vi "Parameter.vi"(9 "In":string, 10 "VIId":string, 11 "VariablesRef":T1) -> ()   [LabVIEW 2018, in "Dialog.lvlib"]
uses:
  Dialog.lvlib
  <userlib>/_OpenG.lib/dictionary/dictionary.llb/Dictionary Object RefNum__ogtk.ctl
  <userlib>/_OpenG.lib/dictionary/dictionary.llb/Dictionary Object RefNum - Enum__ogtk.ctl
  <vilib>/addons/_JKI.lib/Serialization/JSON/JKI JSON Serialization.lvlib
panel:
  in  "Tab Control":enum32{"Config", "控件"}(tab)
  in  "ArrayType":enum32{"AlertDialog", "ConfirmDialog"}(tab)
  in  "对话框文本_AlertDialog":string caption="对话框文本"
  in  "图片名称_AlertDialog":string(combo) caption="图片名称(Config\\Pictures)"
  in  "对话框文本_ConfirmDialog":string caption="对话框文本"
  in  "图片名称_ConfirmDialog":string(combo) caption="图片名称(Config\\Pictures)"
  in  "方法(Method)":enum16{"AlertDialog", "ConfirmDialog"}(ring)
  # "注：图片名称为空，则不显示图片"
  # "注：图片名称为空，则不显示图片"
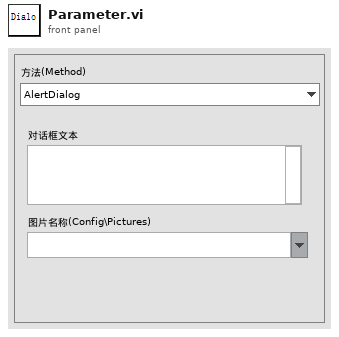
[diagram p1: front panel]
types:
  T1 = typedef "Dictionary Object RefNum__ogtk.ctl" = refnum<k1>
  T2 = cluster{"AlertDialog":cluster{"json":cluster{"Method":string, "Message":string, "PicName":string}}, "ConfirmDialog":cluster{"json":cluster{"Method":string, "Message":string, "PicName":string}}}
  T3 = enum32{"Invalid", "Standard", "Closed", "Hidden", "Minimized", "Maximized"}
  T4 = enum32{"invalid app kind", "Development System", "Run Time System", "Student Edition", "Embedded LabVIEW", "Evaluation", "Custom"}
  T5 = cluster{"Core":cluster{"Current VI Reference":refnum<vi>, "Close Panel on Exit?":bool}, "Parameter":cluster{"VariableRef":T1}, "Synchronize":cluster{"EnqueueData":cluster{"Action":enum16{"Create", "Query", "Revert", "UpdateVariable", "Close"}, "Data":variant}, "Echo":cluster{"VIRef":refnum<vi>, "JsonOut":string, "Status":string}, "Communicate":cluster{"ID":string, "JsonIn":string, "VarRef":T1}, "Queue":refnum<queue>}, "DialogClusters":cluster{"AlertDialog":cluster{"json":cluster{"Method":string, "Message":string, "PicName":string}}, "ConfirmDialog":cluster{"json":cluster{"Method":string, "Message":string, "PicName":string}}}}
  T6 = cluster{"EnqueueData":cluster{"Action":enum16{"Create", "Query", "Revert", "UpdateVariable", "Close"}, "Data":variant}, "Echo":cluster{"VIRef":refnum<vi>, "JsonOut":string, "Status":string}, "Communicate":cluster{"ID":string, "JsonIn":string, "VarRef":T1}, "Queue":refnum<queue>}
  T7 = cluster{"Current VI Reference":refnum<vi>, "Close Panel on Exit?":bool}
  T8 = cluster{"json":cluster{"Method":string, "Message":string, "PicName":string}}
  T9 = cluster{"Action":enum16{"Create", "Query", "Revert", "UpdateVariable", "Close"}, "Data":variant}
  T10 = cluster{"ID":string, "JsonIn":string, "VarRef":T1}
  T11 = enum16{"Create", "Query", "Revert", "UpdateVariable", "Close"}
  T12 = cluster{"VIRef":refnum<vi>, "JsonOut":string, "Status":string}
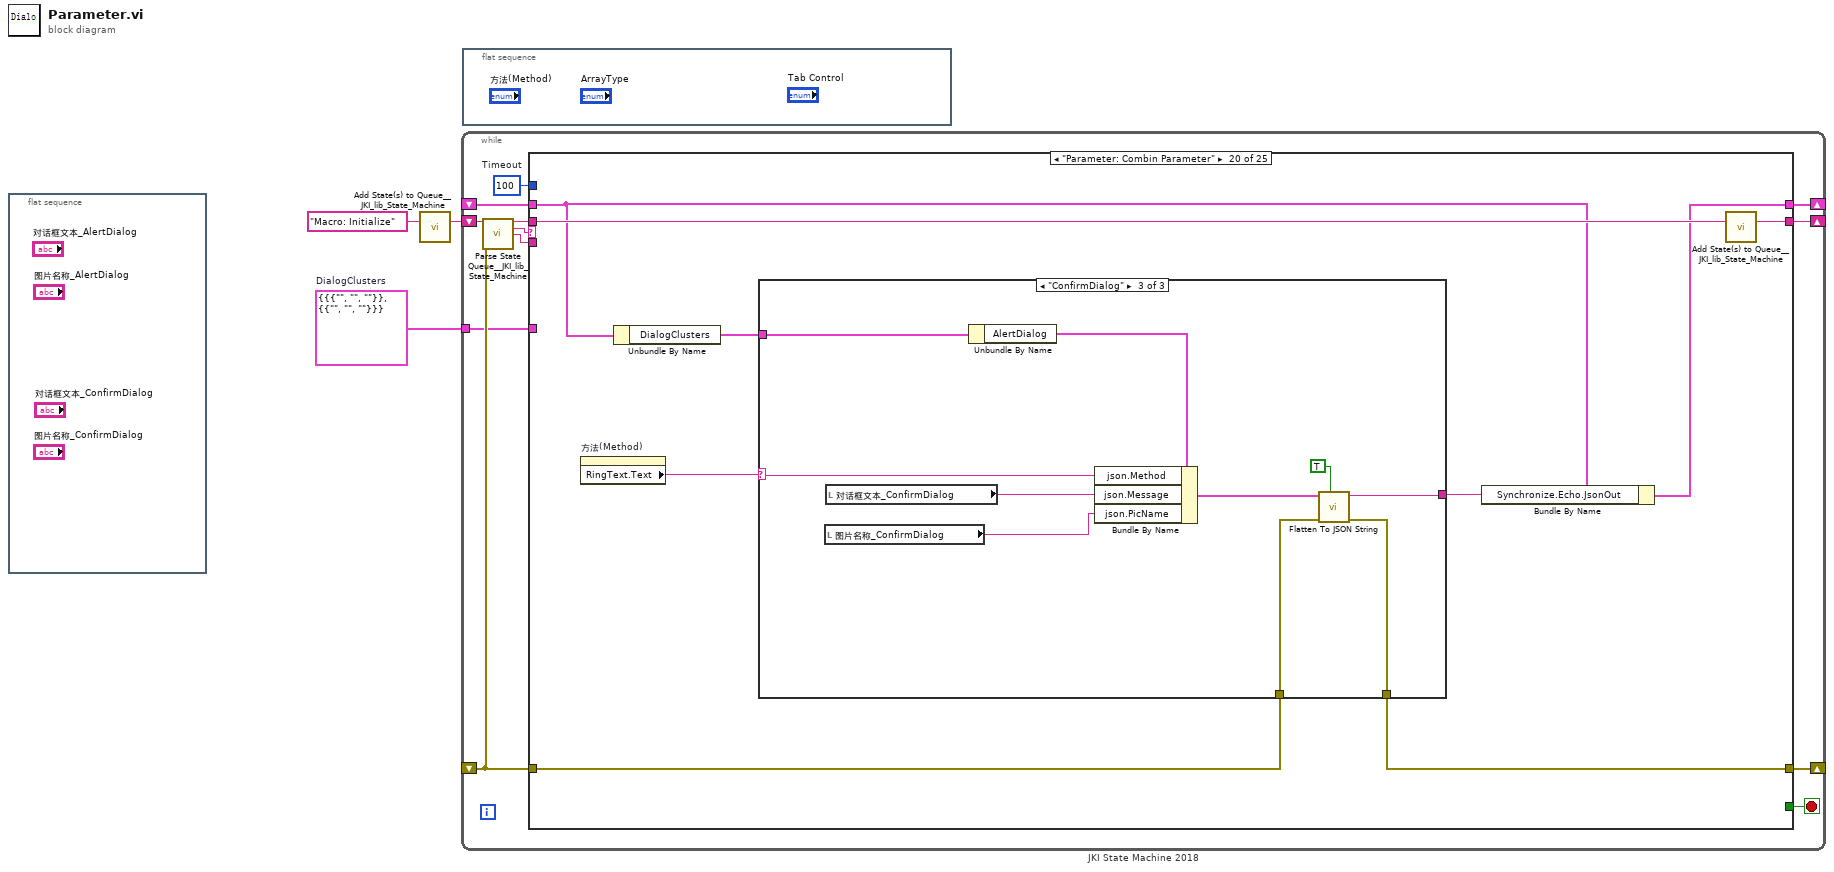
[diagram p0: block diagram]
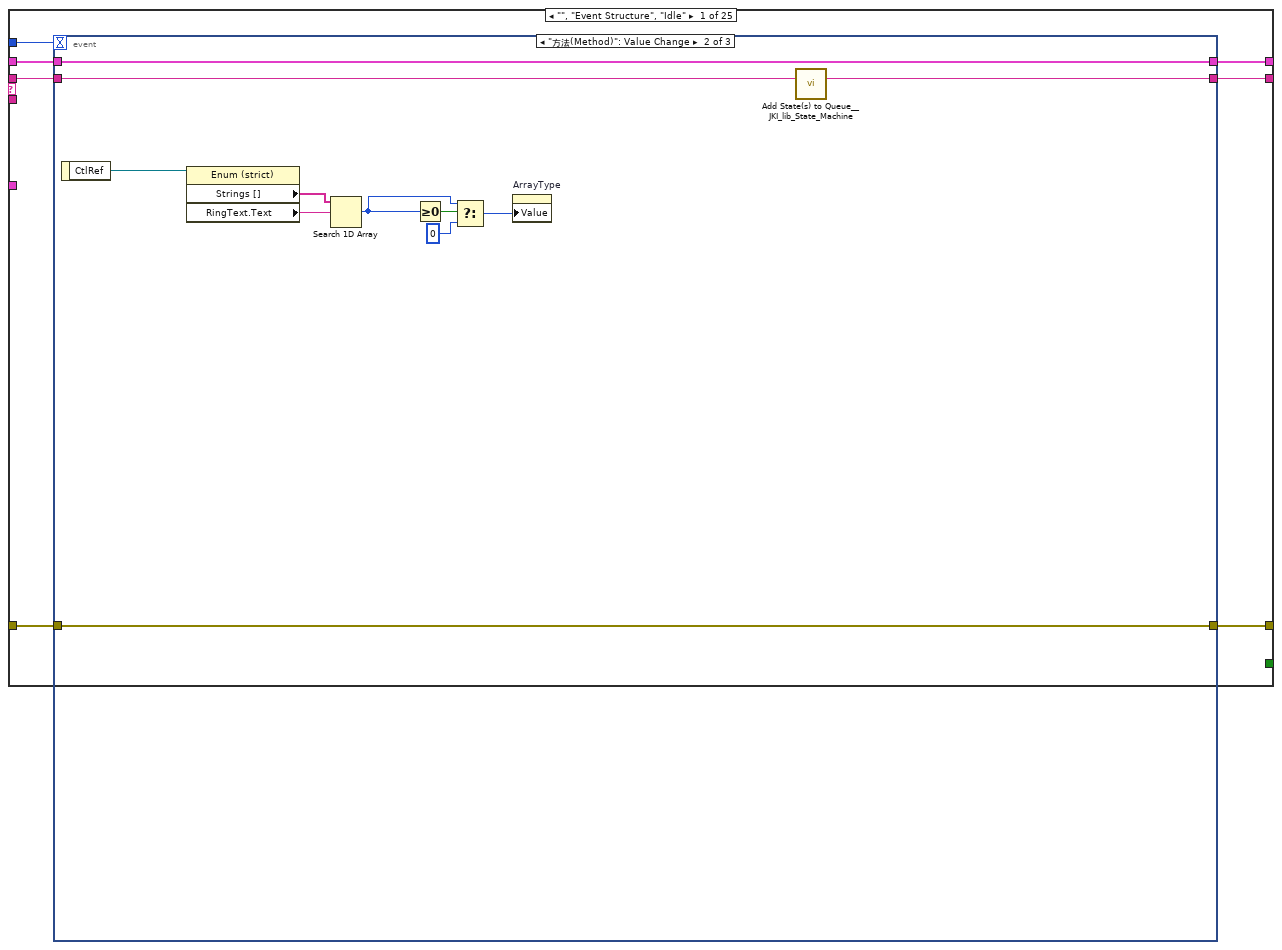
[diagram p2: hidden frame]
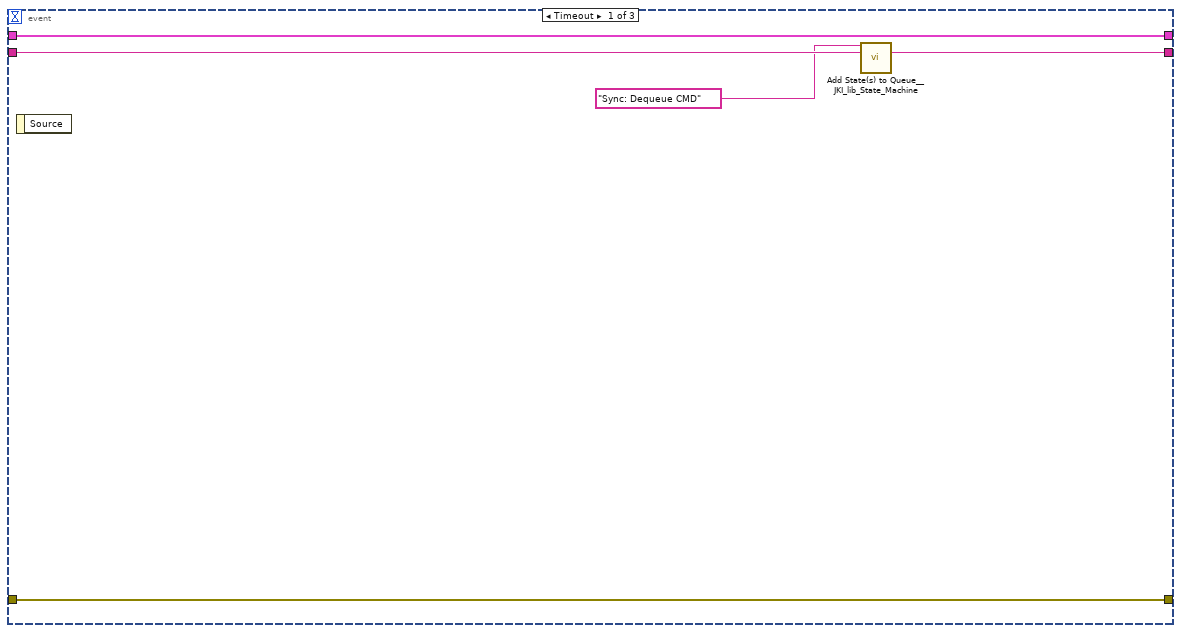
[diagram p3: hidden frame]
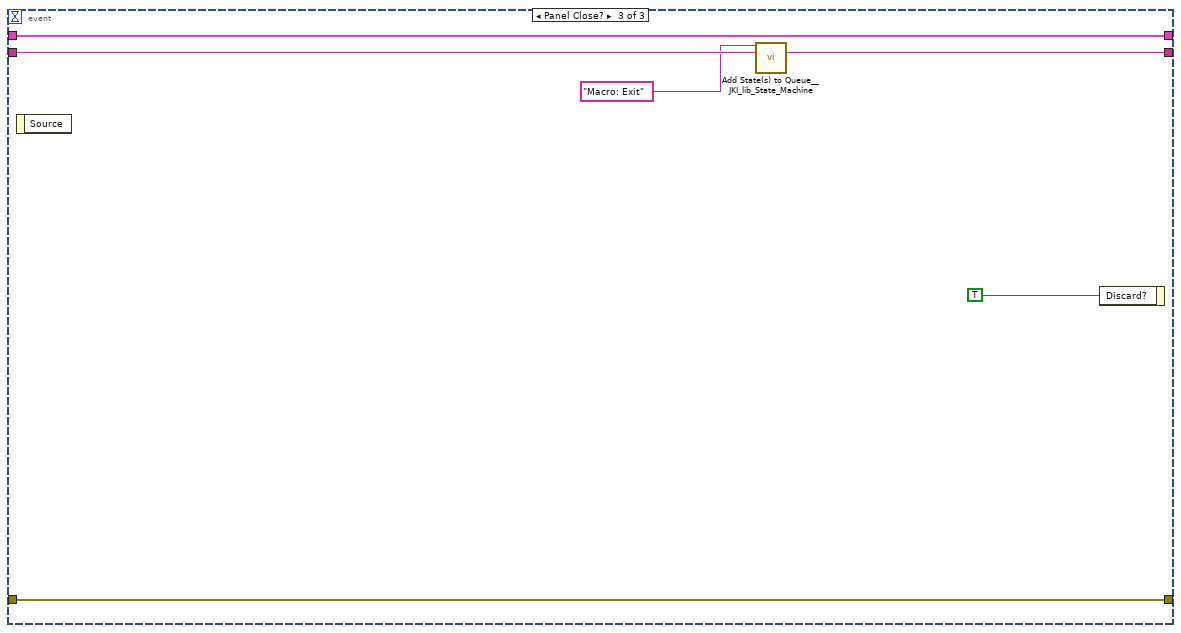
[diagram p4: hidden frame]
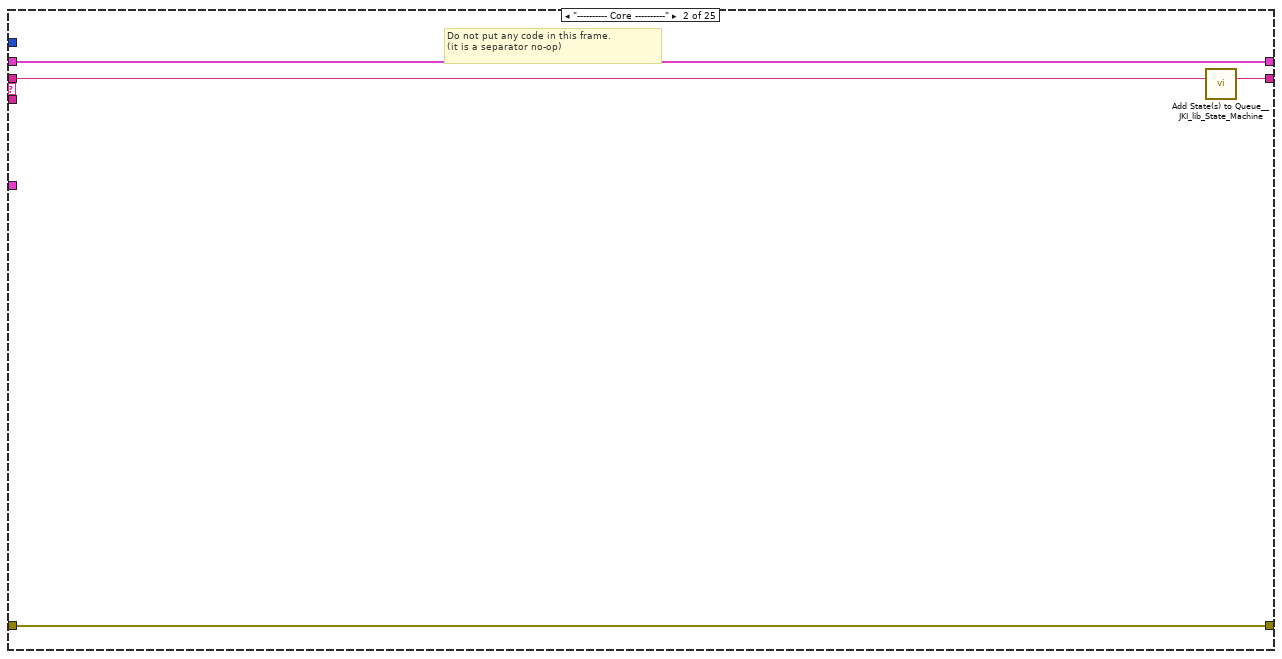
[diagram p5: hidden frame]
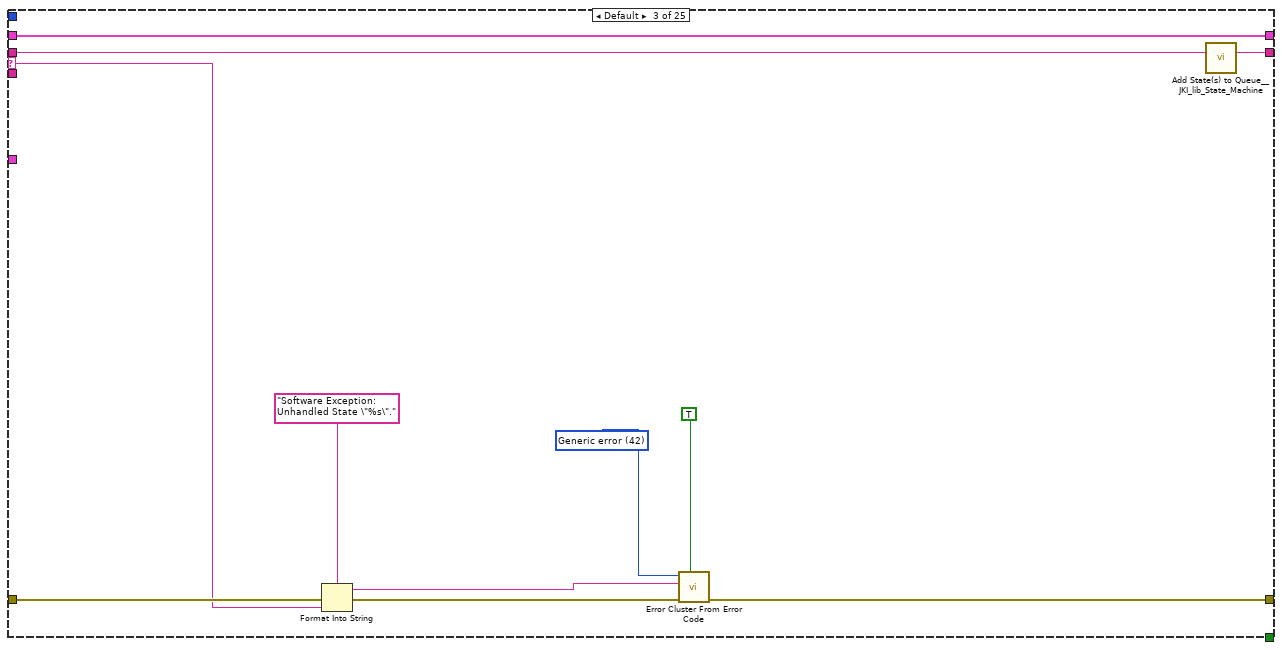
[diagram p6: hidden frame]
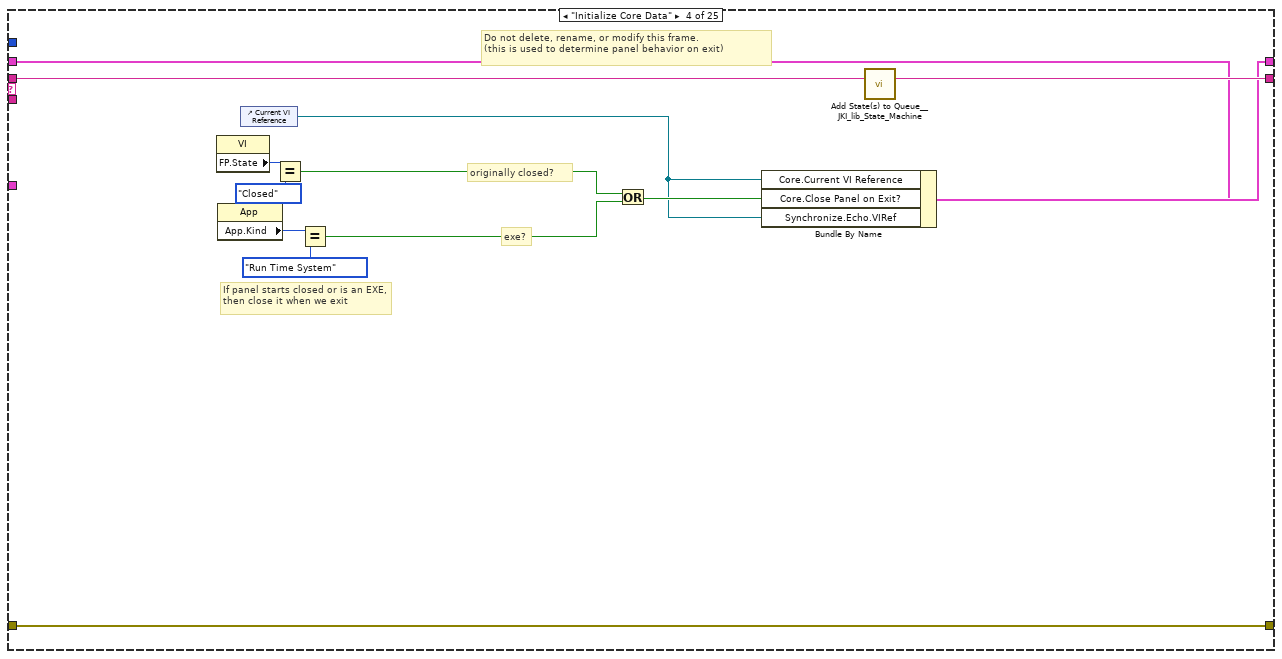
[diagram p7: hidden frame]
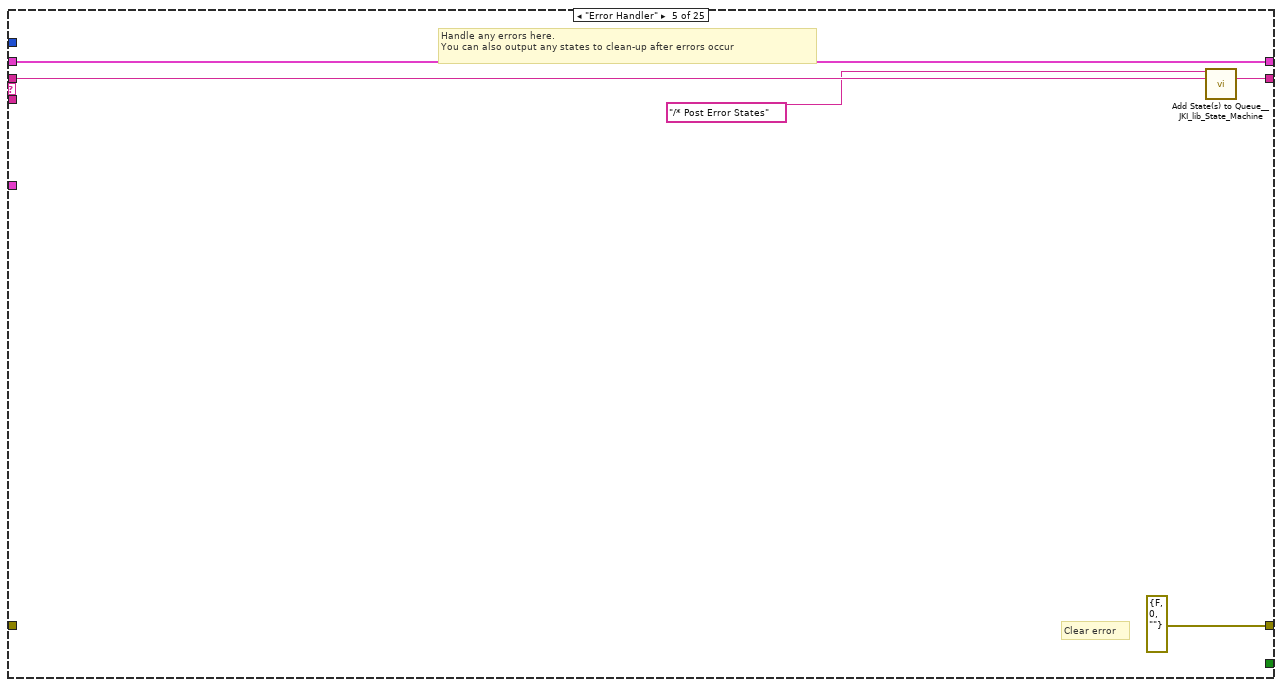
[diagram p8: hidden frame]
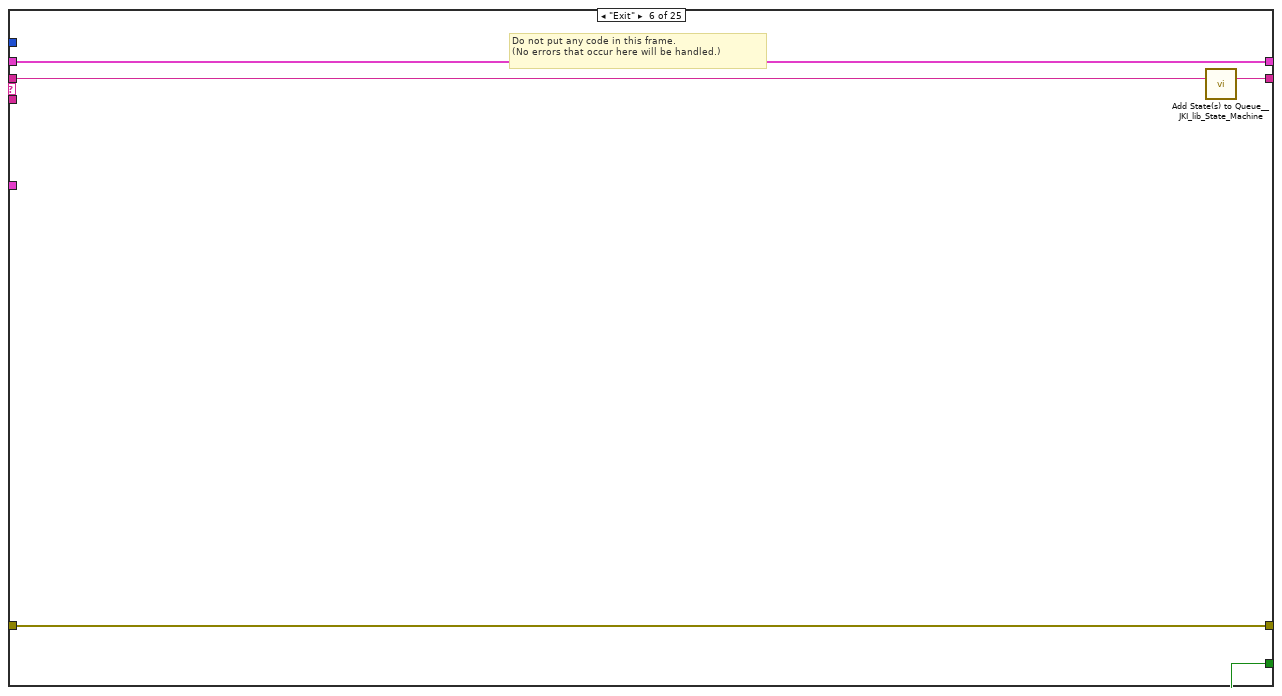
[diagram p9: hidden frame]
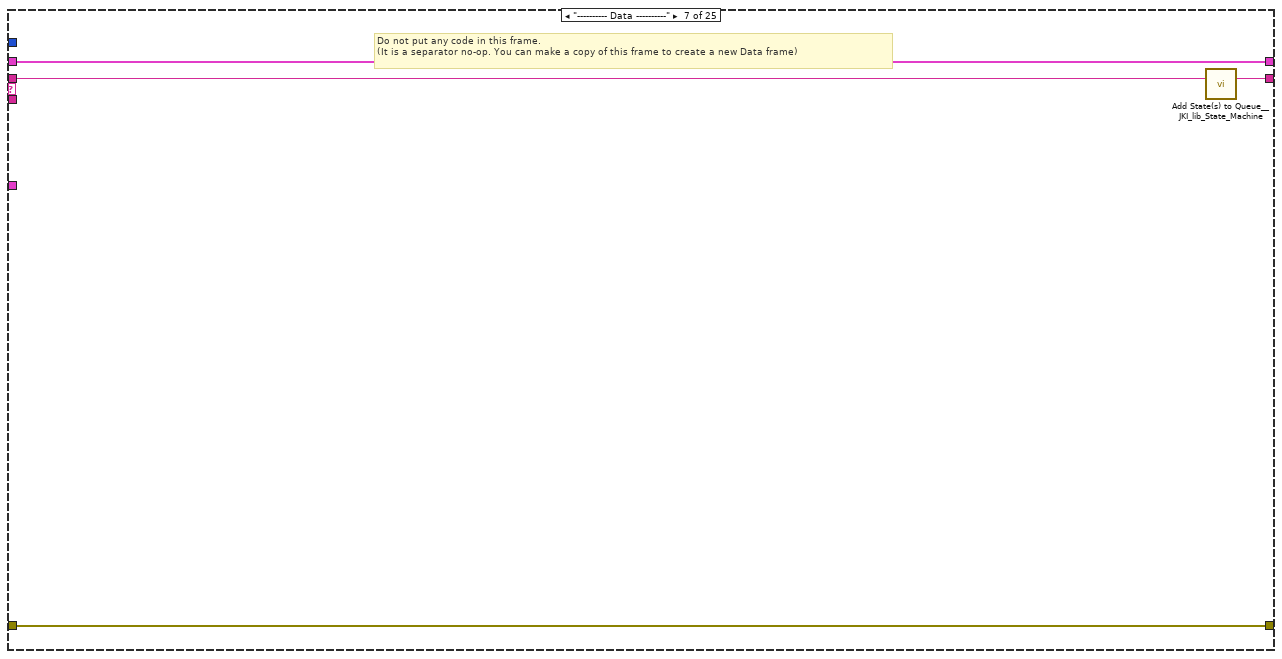
[diagram p10: hidden frame]
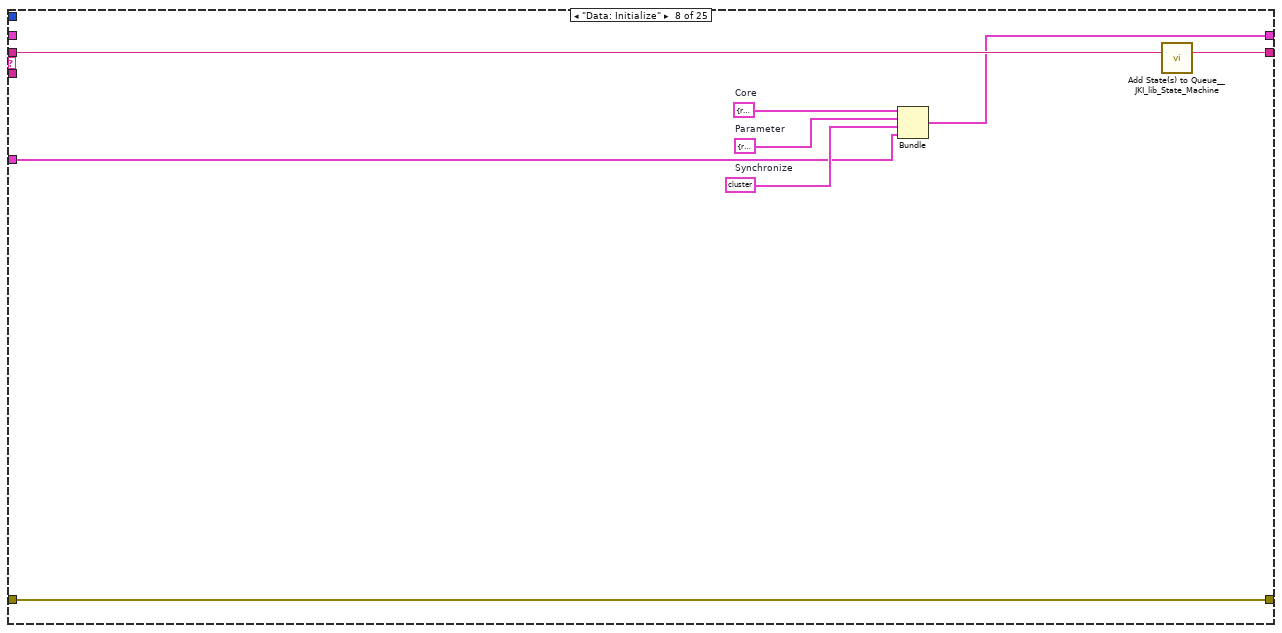
[diagram p11: hidden frame]
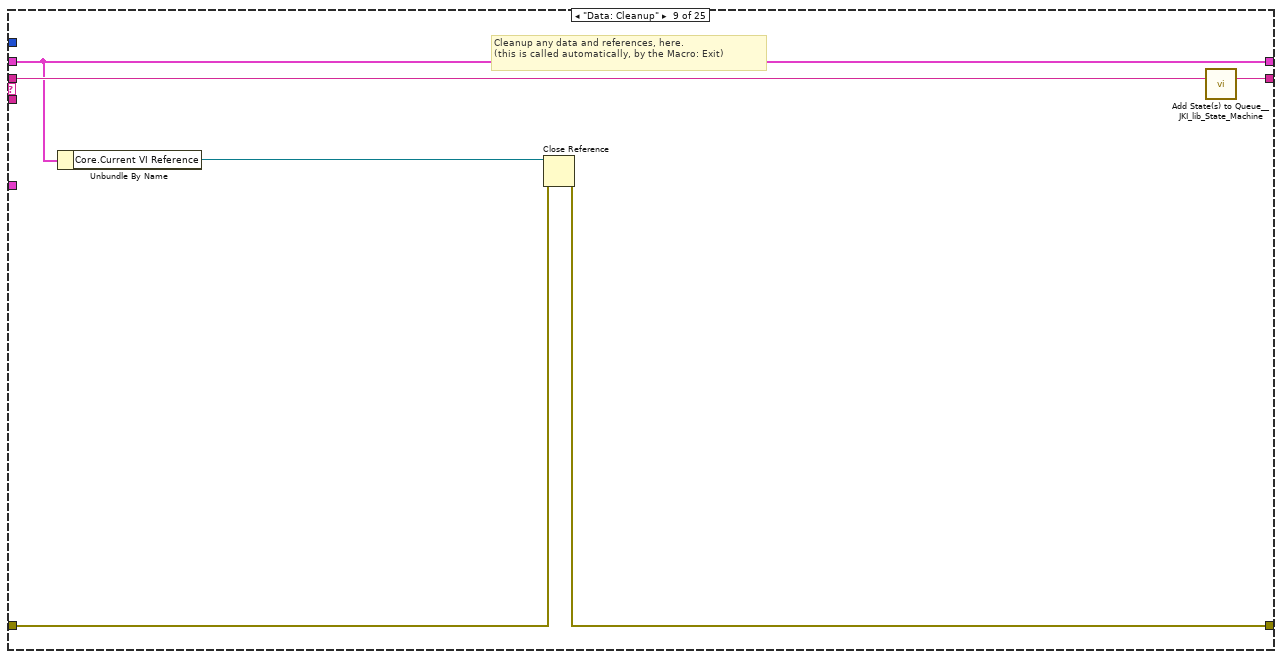
[diagram p12: hidden frame]
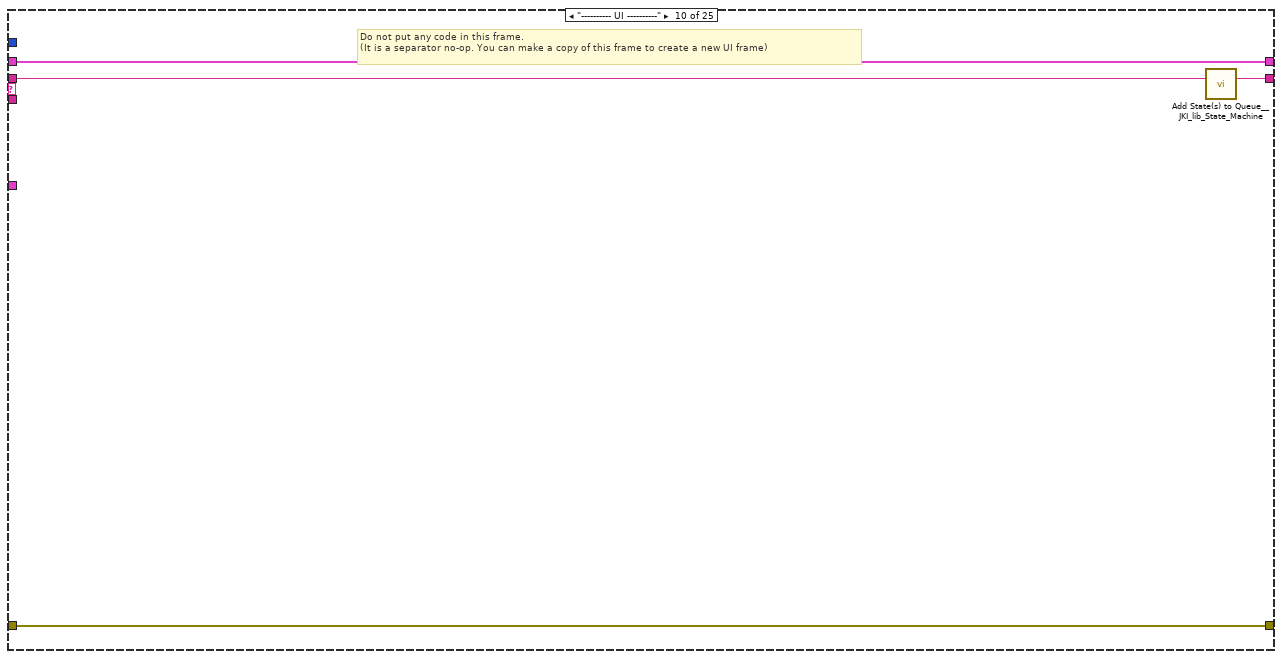
[diagram p13: hidden frame]
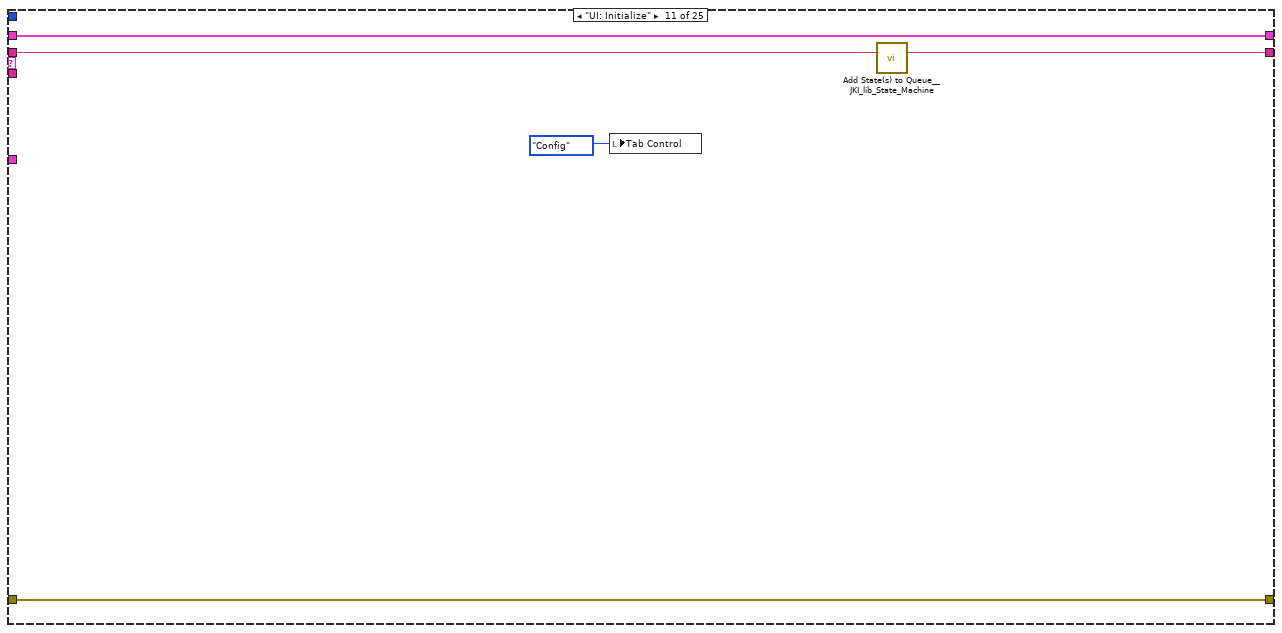
[diagram p14: hidden frame]
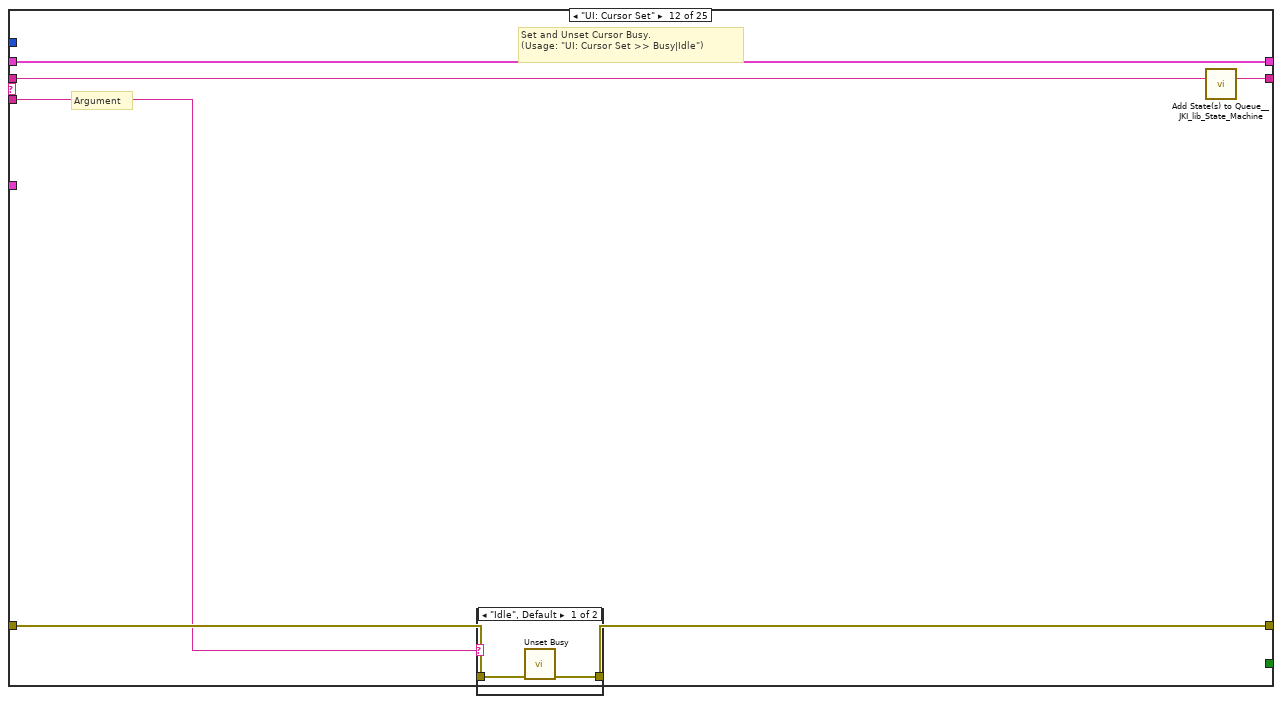
[diagram p15: hidden frame]
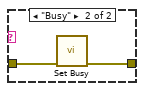
[diagram p16: hidden frame]
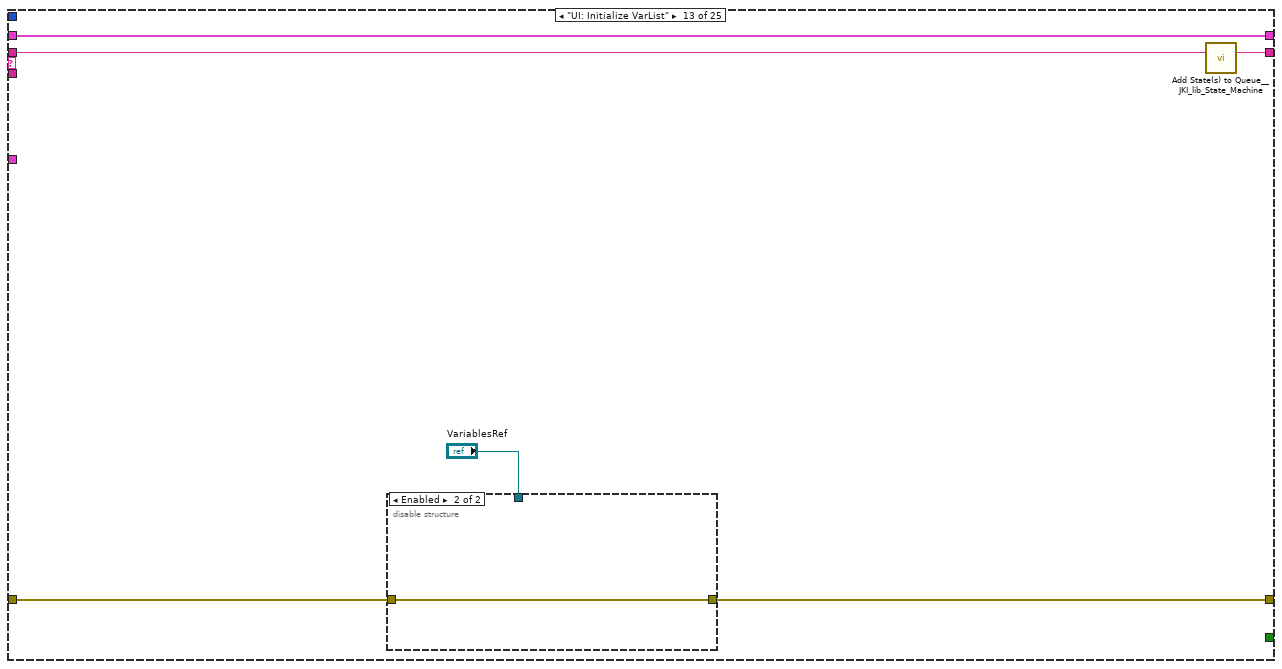
[diagram p17: hidden frame]
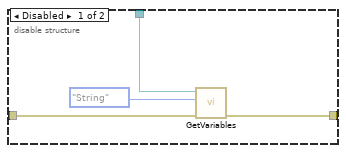
[diagram p18: hidden frame]
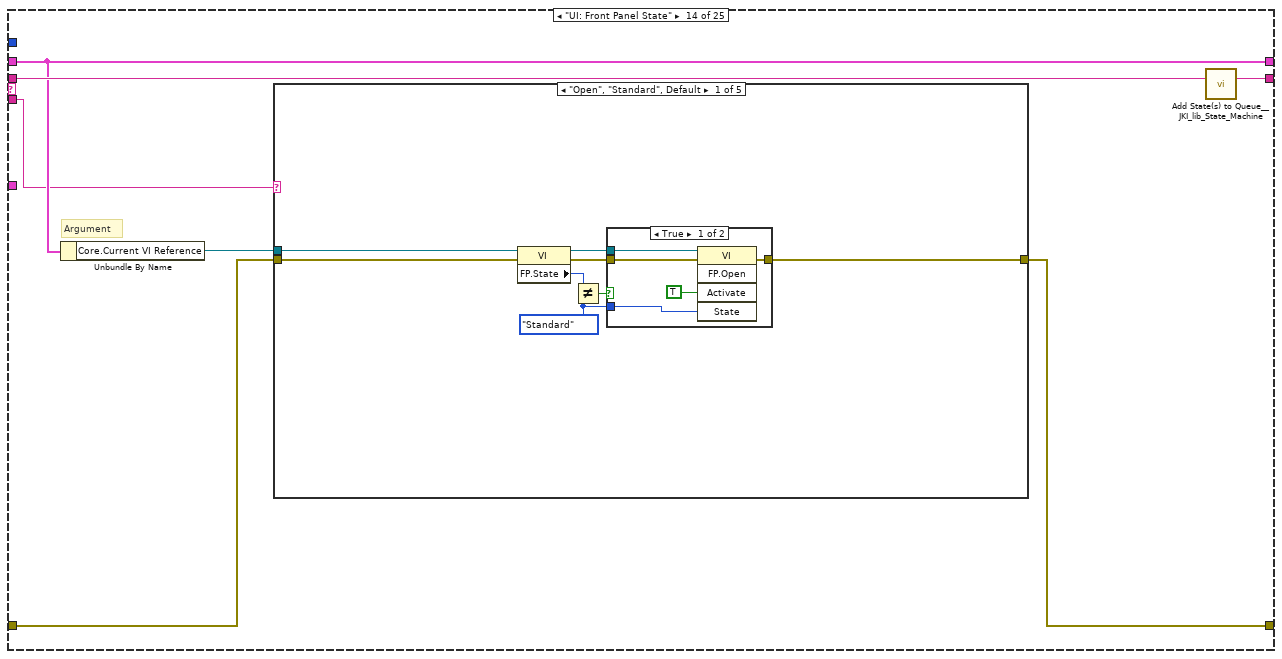
[diagram p19: hidden frame]
diagram:
  w1 = T2 {"AlertDialog"={"json"={"Method"="", "Message"="", "PicName"=""}}, "ConfirmDialog"={"json"={"Method"="", "Message"="", "PicName"=""}}}  # DialogClusters
  n1 = flat-sequence {
    frame #0 {
    }
  }
  n2 = call <vilib>:"Add State(s) to Queue__JKI_lib_State_Machine.vi"("State(s) in (\"\")"="Macro: Initialize") -> ("States Out"=w3:string)  [unwired: 14 in]
  n3 = while "JKI State Machine 2018" {
    shift-right: [w8] -> _
    shift-left: _ -> [w7]
    shift-right: [w11] -> _
    shift-left: _ -> [w5]
    shift-right: [w10] -> _
    shift-left: w3 -> [w12]
    tunnel: w1 -> [w4]
    stop <- w9 stop-if-true
    w6 = 100  # Timeout
    n4 = call <vilib>:"Parse State Queue__JKI_lib_State_Machine.vi"("State Queue"=w12, "Error In (no error)"=w5) -> ("Remaining States"=w14:string, "Current State"=w15:string, "Arguments"=w13:string)  [unwired: 11 in]
    n5 = case shown="\"Parameter: Combin Parameter\"" w15 {
      selector: w15 -> [_ _ w49 _ _ _ _ _ _ _ _ _ _ _ _ _ _ _ _ _ _ _ _ _ _]
      tunnel: w14 -> [w22 w48 w53 w72 w77 w82 w86 w94 w100 w104 w109 w115 w125 w137 w206 w211 w221 w225 w233 w280 w305 w314 w329 w373 w388]
      tunnel: w13 -> [_ _ _ _ _ _ _ _ _ _ _ w110 _ w131 _ _ _ _ _ _ _ _ _ _ _]
      tunnel: w7 -> [w20 w45 w51 w65 w74 w80 w83 _ w95 w101 w106 w113 w123 w133 w203 w208 w218 w222 w228 w273 w302 w307 w327 w370 w377]
      tunnel: [w19 w46 w55 w69 errorcluster {"status"=FALSE, "code"=0, "source"=""} ("error out") w79 w84 w92 w96 w102 w105 w111 w120 w134 w204 w209 w219 w223 w229 w277 w303 w311 w316 w368 w375] -> w11
      tunnel: w5 -> [w18 w46 w54 w69 _ w79 w84 w92 w97 w102 w105 w112 w121 w135 w204 w209 w219 w223 w230 w276 w303 w312 w325 w369 w376]
      tunnel: [w21 w47 w52 w71 w76 w81 w85 w93 w99 w103 w108 w114 w124 w136 w205 w210 w220 w224 w232 w279 w304 w313 w328 w372 w387] -> w10
      tunnel: [_ _ _ _ _ TRUE _ _ _ _ _ _ _ _ _ _ _ _ _ _ _ _ _ _ _] -> w9
      tunnel: [w17 w45 w51 w70 w74 w80 w83 w89 w95 w101 w106 w113 w123 w133 w203 w208 w218 w222 w228 w278 w302 w309 w318 w370 w377] -> w8
      tunnel: w6 -> [w16 _ _ _ _ _ _ _ _ _ _ _ _ _ _ _ _ _ _ _ _ _ _ _ _]
      tunnel: w4 -> [_ _ _ _ _ _ _ w87 _ _ _ _ _ _ _ _ _ _ _ _ _ _ _ _ _]
      frame "", "Event Structure", "Idle" {
        n6 = event shown="[1] \"方法(Method)\": Value Change" {
          selector: _ -> [_ _ _]
          dyn-events: _ -> [_ _ _]
          timeout: w16 -> [_ _ _]
          tunnel: w22 -> [w27 w38 w44]
          tunnel: [w26 w37 w43] -> w21
          tunnel: w20 -> [w24 w35 w41]
          tunnel: [w25 w36 w42] -> w19
          tunnel: w18 -> [w25 w36 w42]
          tunnel: [w24 w35 w41] -> w17
          event Timeout {
            n7 = event-data() -> ()  [unwired: 1 in, 1 out]
            n8 = call <vilib>:"Add State(s) to Queue__JKI_lib_State_Machine.vi"("State(s) in Front (\"\")"="Sync: Dequeue CMD" ("State(s) in Front (\"\")"), "State(s) in (\"\")"=w27) -> ("States Out"=w26:string)  [unwired: 13 in]
          }
          event "方法(Method)": Value Change {
            n9 = event-data() -> ("CtlRef"=w31:refnum<vi>)  [unwired: 1 in]
            n10 = property class="Enum (strict)"(reference=w31) -> ("Strings []"=w30:string[], "RingText.Text"=w29:string)  [unwired: 1 in, 2 out]
            n11 = Search 1D Array(1D array=w30, element=w29) -> (index of element=w33:i32)  [unwired: 1 in]
            n12 = Greater Or Equal To 0?(x=w33) -> (x >= 0?=w34:bool)
            n13 = Select(t=w33, s=w34, f=0) -> (s? t:f=w28:i32)
            n14 = property on="ArrayType" class="TabCtl (strict)"("Value"=w28) -> ()  [unwired: 2 in, 2 out]
            n15 = call <vilib>:"Add State(s) to Queue__JKI_lib_State_Machine.vi"("State(s) in (\"\")"=w38) -> ("States Out"=w37:string)  [unwired: 14 in]
          }
          event Panel Close? {
            n16 = event-data() -> ()  [unwired: 1 in, 1 out]
            n17 = call <vilib>:"Add State(s) to Queue__JKI_lib_State_Machine.vi"("State(s) in Front (\"\")"="Macro: Exit", "State(s) in (\"\")"=w44) -> ("States Out"=w43:string)  [unwired: 13 in]
            n18 = event-data("Discard?"=TRUE) -> ()  [unwired: 1 in, 1 out]
          }
        }
      }
      frame "---------- Core ----------" {
        # "Do not put any code in this frame.\n(it is a separator no-op)"
        n19 = call <vilib>:"Add State(s) to Queue__JKI_lib_State_Machine.vi"("State(s) in (\"\")"=w48) -> ("States Out"=w47:string)  [unwired: 14 in]
      }
      frame Default {
        w58 = 42 items=["No error", "Argument error", "Memory is full", "Out of zone", "End of file", "File already open", "Generic file I/O error", "File not found", "File permission error", "Disk is full", "Duplicate path", "Too many files open", "System feature not enabled", "Resource file not found", "Cannot add resource", "Resource not found", "Image not found", "Image memory error", "Pen does not exist", "Config type invalid", "Config token not found", "Config parse error", "Config memory error", "Bad external code format", "Bad external code offset", "External code not present", "Null window", "Destroy window error", "Null menu", "Print aborted", "Bad print record", "Print driver error", "Windows error during printing", "Memory error during printing", "Print dialog error", "Generic print error", "Invalid device refnum", "Device not found", "Device parameter error", "Device unit error", "Cannot open device", "Device call aborted", "Generic error", "Cancelled by user", "Object ID too low", "Object ID too high", "Object not in heap", "Unknown heap", "Unknown object (invalid DefProc)", "Unknown object (DefProc not in table)", "Message out of range", "Invalid (null) method", "Unknown message", "Manager call not supported", "Bad address", "Network operation in progress", "Network operation timed out", "Connection is busy", "Network attribute not supported", "Network error", "Address in use", "System out of memory", "Connection aborted", "Connection refused", "Not connected", "Already connected", "Connection closed", "Initialization error (interapplication manager)", "Bad occurrence", "Wait on unbound occurrence handler", "Occurrence queue overflow", "Datalog type conflict", "Unused", "Unrecognized type (interapplication manager)", "Memory corrupt", "Failed to make temporary DLL", "Old CIN version", "Drag socket not found", "Failed to load drop-object", "Failed to register OLE object", "Failed to release OLE object", "Format specifier type mismatch", "Unknown format specifier", "Too few format specifiers", "Too many format specifiers", "Scan failed", "Newer CIN version", "Error converting to variant", "Runtime menu error", "Password tampered", "Variant attribute not found", "Incompatible variant data type", "Event data is not available", "Event Store is not present", "Occurrence is not found", "Event Queue is not created", "Event info is not available", "Refnum passed is NULL", "Error retrieving Class GUID", "Error retrieving CoClass GUID", "Error retrieving TypeLib GUID.", "Bad built application magic bytes.", "Specific driver is different from the specific driver associated with the Logical Name.", "There is no session opened to the class driver.", "Max Error", "MAX - Error with config objects", "MAX - Error loading configuration", "MAX - Group not supported"]
        n20 = Format Into String(format string="Software Exception: Unhandled State \"%s\"." ("message"), error in=w54, w49) -> (resulting string=w57:string, error out=w56:errorcluster)  [unwired: 1 in]
        n21 = call <vilib>:"Error Cluster From Error Code.vi"("show call chain? (False)"=TRUE, "error in (no error)"=w56, "error message (\"\")"=w57, "error code (0)"=w58) -> ("error out"=w55:errorcluster)  [unwired: 5 in]
        n22 = call <vilib>:"Add State(s) to Queue__JKI_lib_State_Machine.vi"("State(s) in (\"\")"=w53) -> ("States Out"=w52:string)  [unwired: 14 in]
      }
      frame "Initialize Core Data" {
        # "Do not delete, rename, or modify this frame.\n(this is used to determine panel behavior on exit)"
        # "originally closed?"
        # "exe?"
        # "If panel starts closed or is an EXE, then close it when we exit"
        n23 = property class="VI"() -> ("FP.State"=w63:T3)  [unwired: 2 in, 2 out]
        n24 = property class="App"() -> ("App.Kind"=w68:T4)  [unwired: 2 in, 2 out]
        n25 = control-ref of="Current VI Reference"() -> (w60:refnum<vi>)
        n26 = Equal?(x=w63, y=T3."Closed" ("Front Panel Window:State")) -> (x = y?=w61:bool)
        n27 = Equal?(x=w68, y=T4."Run Time System" ("Application:Kind")) -> (x = y?=w66:bool)
        n28 = Or(x=w61, y=w66) -> (x .or. y?=w64:bool)
        n29 = Bundle By Name(cluster=w65, "Core.Current VI Reference"=w60, "Core.Close Panel on Exit?"=w64, "Synchronize.Echo.VIRef"=w60) -> (w70:T5)
        n30 = call <vilib>:"Add State(s) to Queue__JKI_lib_State_Machine.vi"("State(s) in (\"\")"=w72) -> ("States Out"=w71:string)  [unwired: 14 in]
      }
      frame "Error Handler" {
        # "Handle any errors here.\nYou can also output any states to clean-up after errors occur"
        # "Clear error"
        n31 = call <vilib>:"Add State(s) to Queue__JKI_lib_State_Machine.vi"("State(s) in Front (\"\")"="/* Post Error States", "State(s) in (\"\")"=w77) -> ("States Out"=w76:string)  [unwired: 13 in]
      }
      frame "Exit" {
        # "Do not put any code in this frame.\n(No errors that occur here will be handled.)"
        n32 = call <vilib>:"Add State(s) to Queue__JKI_lib_State_Machine.vi"("State(s) in (\"\")"=w82) -> ("States Out"=w81:string)  [unwired: 14 in]
      }
      frame "---------- Data ----------" {
        # "Do not put any code in this frame.\n(It is a separator no-op. You can make a copy of this frame to create a new Data frame)"
        n33 = call <vilib>:"Add State(s) to Queue__JKI_lib_State_Machine.vi"("State(s) in (\"\")"=w86) -> ("States Out"=w85:string)  [unwired: 14 in]
      }
      frame "Data: Initialize" {
        w88 = cluster{"VariableRef":T1} {"VariableRef"=refnum}  # Parameter
        w90 = T6 {"EnqueueData"={"Action"=enum."Create", "Data"=variant}, "Echo"={"VIRef"=refnum, "JsonOut"="", "Status"=""}, "Communicate"={"ID"="", "JsonIn"="", "VarRef"=refnum}, "Queue"=refnum}  # Synchronize
        w91 = T7 {"Current VI Reference"=refnum, "Close Panel on Exit?"=FALSE}  # Core
        n34 = Bundle("Core"=w91, "Parameter"=w88, "Synchronize"=w90, "DialogClusters"=w87) -> (w89:T5)  [unwired: 1 in]
        n35 = call <vilib>:"Add State(s) to Queue__JKI_lib_State_Machine.vi"("State(s) in (\"\")"=w94) -> ("States Out"=w93:string)  [unwired: 14 in]
      }
      frame "Data: Cleanup" {
        # "Cleanup any data and references, here.\n(this is called automatically, by the Macro: Exit)"
        n36 = Unbundle By Name(w95) -> ("Core.Current VI Reference"=w98:refnum<vi>)
        n37 = Close Reference(reference=w98, error in (no error)=w97) -> (error out=w96:errorcluster)
        n38 = call <vilib>:"Add State(s) to Queue__JKI_lib_State_Machine.vi"("State(s) in (\"\")"=w100) -> ("States Out"=w99:string)  [unwired: 14 in]
      }
      frame "---------- UI ----------" {
        # "Do not put any code in this frame.\n(It is a separator no-op. You can make a copy of this frame to create a new UI frame)"
        n39 = call <vilib>:"Add State(s) to Queue__JKI_lib_State_Machine.vi"("State(s) in (\"\")"=w104) -> ("States Out"=w103:string)  [unwired: 14 in]
      }
      frame "UI: Initialize" {
        n40 = local write "Tab Control"(enum32{"Config", "控件"}."Config" ("Tab Control")) -> ()
        n41 = call <vilib>:"Add State(s) to Queue__JKI_lib_State_Machine.vi"("State(s) in (\"\")"=w109) -> ("States Out"=w108:string)  [unwired: 14 in]
      }
      frame "UI: Cursor Set" {
        # "Argument"
        # "Set and Unset Cursor Busy.\n(Usage: \"UI: Cursor Set >> Busy|Idle\")"
        n42 = case shown="\"Idle\", Default" w110 {
          tunnel: w112 -> [w117 w119]
          tunnel: [w116 w118] -> w111
          frame "Idle", Default {
            n43 = call <vilib>:"Unset Busy.vi"("error in (no error)"=w117) -> ("error out"=w116:errorcluster)  [unwired: 10 in]
          }
          frame "Busy" {
            n44 = call <vilib>:"Set Busy.vi"("error in (no error)"=w119) -> ("error out"=w118:errorcluster)  [unwired: 9 in, 1 out]
          }
        }
        n45 = call <vilib>:"Add State(s) to Queue__JKI_lib_State_Machine.vi"("State(s) in (\"\")"=w115) -> ("States Out"=w114:string)  [unwired: 14 in]
      }
      frame "UI: Initialize VarList" {
        n46 = disable-structure shown="Enabled" {
          disable-tunnel: "VariablesRef" -> [w129 _]
          disable-tunnel: w121 -> [w127 w130]
          disable-tunnel: [w126 w130] -> w120
          frame Disabled {
            n47 = call "GetVariables.vi"("error in (no error)"=w127, "VariableType"=enum16{"String", "StringArray"}."String", "DicRef"=w129) -> ("error out"=w126:errorcluster)  [unwired: 7 in, 1 out]
          }
          frame Enabled {
          }
        }
        n48 = call <vilib>:"Add State(s) to Queue__JKI_lib_State_Machine.vi"("State(s) in (\"\")"=w125) -> ("States Out"=w124:string)  [unwired: 14 in]
      }
      frame "UI: Front Panel State" {
        # "Argument"
        n49 = Unbundle By Name(w133) -> ("Core.Current VI Reference"=w132:refnum<vi>)
        n50 = case shown="\"Open\", \"Standard\", Default" w131 {
          tunnel: w135 -> [w143 w158 w169 w182 w195]
          tunnel: [w145 w159 w171 w184 w197] -> w134
          tunnel: w132 -> [w144 w156 w170 w183 w196]
          frame "Open", "Standard", Default {
            w138 = T3."Standard" ("State")
            n51 = property class="VI"(reference=w144, error in=w143) -> (reference out=w141:refnum<vi>, error out=w142:errorcluster, "FP.State"=w140:T3)
            n52 = Not Equal?(x=w140, y=w138) -> (x != y?=w139:bool)
            n53 = case shown="True" w139 {
              tunnel: [w149 w151] -> w145
              tunnel: w142 -> [w148 w151]
              tunnel: w141 -> [w147 _]
              tunnel: w138 -> [w146 _]
              frame True {
                n54 = invoke class="VI" method="FP.Open"(reference=w147, error in=w148, "Activate"=TRUE, "State"=w146) -> (error out=w149:errorcluster)  [unwired: 1 in, 4 out]
              }
              frame False {
              }
            }
          }
          frame "Close", "Closed" {
            n55 = property class="VI"(reference=w156, error in=w158) -> (reference out=w155:refnum<vi>, error out=w157:errorcluster, "FP.State"=w153:T3)
            n56 = Not Equal?(x=w153, y=T3."Closed" ("Front Panel Window:State")) -> (x != y?=w152:bool)
            n57 = case shown="True" w152 {
              tunnel: [w160 w163] -> w159
              tunnel: w157 -> [w160 w162]
              tunnel: w155 -> [_ w161]
              frame False {
              }
              frame True {
                n58 = invoke class="VI" method="FP.Close"(reference=w161, error in=w162) -> (error out=w163:errorcluster)  [unwired: 1 in, 2 out]
              }
            }
          }
          frame "Hidden", "Hide" {
            w164 = T3."Hidden" ("State")
            n59 = property class="VI"(reference=w170, error in=w169) -> (reference out=w167:refnum<vi>, error out=w168:errorcluster, "FP.State"=w166:T3)
            n60 = Not Equal?(x=w166, y=w164) -> (x != y?=w165:bool)
            n61 = case shown="True" w165 {
              tunnel: [w175 w176] -> w171
              tunnel: w168 -> [w174 w176]
              tunnel: w167 -> [w173 _]
              tunnel: w164 -> [w172 _]
              frame True {
                n62 = invoke class="VI" method="FP.Open"(reference=w173, error in=w174, "State"=w172) -> (error out=w175:errorcluster)  [unwired: 2 in, 4 out]
              }
              frame False {
              }
            }
          }
          frame "Minimize", "Minimized" {
            w177 = T3."Minimized" ("State")
            n63 = property class="VI"(reference=w183, error in=w182) -> (reference out=w180:refnum<vi>, error out=w181:errorcluster, "FP.State"=w179:T3)
            n64 = Not Equal?(x=w179, y=w177) -> (x != y?=w178:bool)
            n65 = case shown="True" w178 {
              tunnel: [w188 w189] -> w184
              tunnel: w181 -> [w187 w189]
              tunnel: w180 -> [w186 _]
              tunnel: w177 -> [w185 _]
              frame True {
                n66 = invoke class="VI" method="FP.Open"(reference=w186, error in=w187, "State"=w185) -> (error out=w188:errorcluster)  [unwired: 2 in, 4 out]
              }
              frame False {
              }
            }
          }
          frame "Maximize", "Maximized" {
            w190 = T3."Maximized" ("State")
            n67 = property class="VI"(reference=w196, error in=w195) -> (reference out=w193:refnum<vi>, error out=w194:errorcluster, "FP.State"=w192:T3)
            n68 = Not Equal?(x=w192, y=w190) -> (x != y?=w191:bool)
            n69 = case shown="True" w191 {
              tunnel: [w201 w202] -> w197
              tunnel: w194 -> [w200 w202]
              tunnel: w193 -> [w199 _]
              tunnel: w190 -> [w198 _]
              frame True {
                n70 = invoke class="VI" method="FP.Open"(reference=w199, error in=w200, "State"=w198) -> (error out=w201:errorcluster)  [unwired: 2 in, 4 out]
              }
              frame False {
              }
            }
          }
        }
        n71 = call <vilib>:"Add State(s) to Queue__JKI_lib_State_Machine.vi"("State(s) in (\"\")"=w137) -> ("States Out"=w136:string)  [unwired: 14 in]
      }
      frame "---------- Macro ----------" {
        n72 = call <vilib>:"Add State(s) to Queue__JKI_lib_State_Machine.vi"("State(s) in (\"\")"=w206) -> ("States Out"=w205:string)  [unwired: 14 in]
      }
      frame "Macro: Initialize" {
        n73 = call <vilib>:"Add State(s) to Queue__JKI_lib_State_Machine.vi"("State(s) in Front (\"\")"="Data: Initialize\nInitialize Core Data\nUI: Initialize\nSync: Obtain CMD Queue\nSync: Dequeue CMD\nUI: Initialize VarList\nParameter: Parse Parameter", "State(s) in (\"\")"=w211) -> ("States Out"=w210:string)  [unwired: 13 in]
      }
      frame "Macro: Exit" {
        n74 = Unbundle By Name(w218) -> ("Core.Close Panel on Exit?"=w217:bool)
        n75 = Select(t="UI: Front Panel State >> Close", s=w217, f="") -> (s? t:f=w214:string)
        n76 = call <vilib>:"Add State(s) to Queue__JKI_lib_State_Machine.vi"("State(s) in (\"\")"=w214, "State(s) at Back (\"\")"="Sync: Release CMD Queue\nData: Cleanup\nExit") -> ("States Out"=w212:string)  [unwired: 13 in]
        n77 = call <vilib>:"Add State(s) to Queue__JKI_lib_State_Machine.vi"("State(s) in Front (\"\")"=w212, "State(s) in (\"\")"=w221) -> ("States Out"=w220:string)  [unwired: 13 in]
      }
      frame "---------- Parameter ----------" {
        # "Template Separator\n(You can make a copy of, or modify, this frame)"
        n78 = call <vilib>:"Add State(s) to Queue__JKI_lib_State_Machine.vi"("State(s) in (\"\")"=w225) -> ("States Out"=w224:string)  [unwired: 14 in]
      }
      frame "Parameter: Parse Parameter" {
        n79 = Unbundle By Name(w228) -> ("DialogClusters"=w227:T2)
        n80 = Empty String/Path?(string/path="In") -> (empty?=w231:bool)
        n81 = case shown="False" w231 {
          tunnel: "In" -> [w242 _]
          tunnel: w230 -> [w247 w271]
          tunnel: [w246 w271] -> w229
          tunnel: w227 -> [w245 _]
          frame False {
            n82 = Match Pattern(string=w242, regular expression="\"Method\":\"") -> (after substring=w241:string)  [unwired: 1 in, 3 out]
            n83 = Match Pattern(string=w241, regular expression="\",") -> (before substring=w240:string)  [unwired: 1 in, 3 out]
            n84 = case shown="\"ConfirmDialog\"" w240 {
              tunnel: w242 -> [w256 w267 _]
              tunnel: w247 -> [w254 w265 w270]
              tunnel: [w253 w264 w270] -> w246
              tunnel: w245 -> [w251 w262 _]
              tunnel: [w252 w263 _] -> w235
              frame "AlertDialog" {
                n85 = Unbundle By Name(w251) -> ("AlertDialog"=w250:T8)
                n86 = call <vilib>:"Unflatten From JSON String.vi"("Type and Defaults"=w250, "error in (no error)"=w254, "JSON String"=w256) -> ("error out"=w257:errorcluster, "Variant"=w258:variant)  [unwired: 7 in]
                n87 = Variant To Data(error in=w257, type=w250, Variant=w258) -> (data=w255:T8, error out=w253:errorcluster)
                n88 = Unbundle By Name(w255) -> ("json.Method"=w252:string, "json.Message"=w249:string, "json.PicName"=w248:string)
                n89 = local write "对话框文本_AlertDialog"(w249) -> ()
                n90 = local write "图片名称_AlertDialog"(w248) -> ()
              }
              frame "ConfirmDialog" {
                n91 = Unbundle By Name(w262) -> ("ConfirmDialog"=w261:T8)
                n92 = call <vilib>:"Unflatten From JSON String.vi"("Type and Defaults"=w261, "error in (no error)"=w265, "JSON String"=w267) -> ("error out"=w268:errorcluster, "Variant"=w269:variant)  [unwired: 7 in]
                n93 = Variant To Data(error in=w268, type=w261, Variant=w269) -> (data=w266:T8, error out=w264:errorcluster)
                n94 = Unbundle By Name(w266) -> ("json.Method"=w263:string, "json.Message"=w260:string, "json.PicName"=w259:string)
                n95 = local write "图片名称_ConfirmDialog"(w259) -> ()
                n96 = local write "对话框文本_ConfirmDialog"(w260) -> ()
              }
              frame Default {
              }
            }
            n97 = property on="方法(Method)" class="Enum (strict)"() -> ("Strings []"=w237:string[])  [unwired: 2 in, 2 out]
            n98 = Search 1D Array(1D array=w237, element=w235) -> (index of element=w239:i32)  [unwired: 1 in]
            n99 = Greater Or Equal To 0?(x=w239) -> (x >= 0?=w238:bool)
            n100 = Select(t=w239, s=w238, f=0) -> (s? t:f=w234:i32)
            n101 = local write "ArrayType"(w234) -> ()
            n102 = property on="方法(Method)" class="Enum (strict)"("Value"=w234) -> ()  [unwired: 2 in, 2 out]
          }
          frame True {
          }
        }
        n103 = call <vilib>:"Add State(s) to Queue__JKI_lib_State_Machine.vi"("State(s) in (\"\")"=w233) -> ("States Out"=w232:string)  [unwired: 14 in]
      }
      frame "Parameter: Combin Parameter" {
        n104 = property on="方法(Method)" class="Enum (strict)"() -> ("RingText.Text"=w275:string)  [unwired: 2 in, 2 out]
        n105 = Unbundle By Name(w273) -> ("DialogClusters"=w272:T2)
        n106 = case shown="\"ConfirmDialog\"" w275 {
          selector: w275 -> [_ w285 w295]
          tunnel: w272 -> [_ w291 w301]
          tunnel: [_ w289 w299] -> w274
          tunnel: [w281 w284 w294] -> w277
          tunnel: w276 -> [w281 w287 w297]
          frame Default {
          }
          frame "AlertDialog" {
            n107 = local read "对话框文本_AlertDialog"() -> (w282:string)
            n108 = local read "图片名称_AlertDialog"() -> (w283:string)
            n109 = Unbundle By Name(w291) -> ("AlertDialog"=w290:T8)
            n110 = Bundle By Name(cluster=w290, "json.Method"=w285, "json.Message"=w282, "json.PicName"=w283) -> (w286:T8)
            n111 = call <vilib>:"Flatten To JSON String.vi"("Multiline (T)"=TRUE, "error in (no error)"=w287, "Variant"=w286) -> ("error out"=w284:errorcluster, "JSON String"=w289:string)  [unwired: 7 in]
          }
          frame "ConfirmDialog" {
            n112 = local read "图片名称_ConfirmDialog"() -> (w292:string)
            n113 = local read "对话框文本_ConfirmDialog"() -> (w293:string)
            n114 = Unbundle By Name(w301) -> ("AlertDialog"=w300:T8)
            n115 = Bundle By Name(cluster=w300, "json.Method"=w295, "json.Message"=w293, "json.PicName"=w292) -> (w296:T8)
            n116 = call <vilib>:"Flatten To JSON String.vi"("Multiline (T)"=TRUE, "error in (no error)"=w297, "Variant"=w296) -> ("error out"=w294:errorcluster, "JSON String"=w299:string)  [unwired: 7 in]
          }
        }
        n117 = Bundle By Name(cluster=w273, "Synchronize.Echo.JsonOut"=w274) -> (w278:T5)
        n118 = call <vilib>:"Add State(s) to Queue__JKI_lib_State_Machine.vi"("State(s) in (\"\")"=w280) -> ("States Out"=w279:string)  [unwired: 14 in]
      }
      frame "---------- Sync ----------" {
        n119 = call <vilib>:"Add State(s) to Queue__JKI_lib_State_Machine.vi"("State(s) in (\"\")"=w305) -> ("States Out"=w304:string)  [unwired: 14 in]
      }
      frame "Sync: Obtain CMD Queue" {
        # "这里由平台输入"
        n120 = Unbundle By Name(w307) -> ("Synchronize.EnqueueData"=w306:T9)
        n121 = Obtain Queue(name (unnamed)="VIId", element data type=w306, error in (no error)=w312) -> (queue out=w308:refnum<queue>, error out=w311:errorcluster)  [unwired: 2 in, 1 out]
        n122 = Bundle By Name(cluster=w307, "Synchronize.Queue"=w308) -> (w309:T5)
        n123 = call <vilib>:"Add State(s) to Queue__JKI_lib_State_Machine.vi"("State(s) in (\"\")"=w314) -> ("States Out"=w313:string)  [unwired: 14 in]
      }
      frame "Sync: Dequeue CMD" {
        n124 = Unbundle By Name(w327) -> ("Synchronize.Queue"=w324:refnum<queue>, "Synchronize.Communicate"=w315:T10)
        n125 = Dequeue Element(queue=w324, timeout in ms (-1)=10, error in (no error)=w325) -> (queue out=w323:refnum<queue>, element=w321:T9, timed out?=w322:bool, error out=w317:errorcluster)
        n126 = Bundle By Name(cluster=w327, "Synchronize.Queue"=w323, "Synchronize.EnqueueData"=w321) -> (w319:T5)
        n127 = case shown="False" w322 {
          tunnel: w321 -> [w338 _]
          tunnel: [w336 _] -> w320
          tunnel: w319 -> [w335 w367]
          tunnel: [w334 w367] -> w318
          tunnel: w317 -> [w332 w366]
          tunnel: [w331 w366] -> w316
          tunnel: w315 -> [w330 _]
          frame False {
            n128 = Unbundle By Name(w338) -> ("Action"=w337:T11, "Data"=w333:variant)
            n129 = case shown="\"Query\"" w337 {
              tunnel: ["Sync: Send ECHO" "UI: Initialize VarList\nSync: Send ECHO" _ "Sync: Send ECHO\nMacro: Exit" "Parameter: Combin Parameter\nSync: Send ECHO" "Parameter: Parse Parameter\nSync: Send ECHO"] -> w336
              tunnel: w335 -> [w341 w346 w350 w353 w358 w363]
              tunnel: [w340 w345 w350 w352 w357 w362] -> w334
              tunnel: w333 -> [_ _ _ _ _ _]
              tunnel: w332 -> [w342 w347 w349 w354 w359 w364]
              tunnel: [w342 w347 w349 w354 w359 w364] -> w331
              tunnel: w330 -> [_ _ _ _ _ _]
              frame "Create" {
                n130 = Bundle By Name(cluster=w341, "Synchronize.Echo.Status"="Create Success") -> (w340:T5)
              }
              frame "UpdateVariable" {
                n131 = Bundle By Name(cluster=w346, "Synchronize.Echo.Status"="UpdateVariable Success") -> (w345:T5)
              }
              frame Default {
              }
              frame "Close" {
                n132 = Bundle By Name(cluster=w353, "Synchronize.Echo.Status"="Close Success") -> (w352:T5)
              }
              frame "Query" {
                n133 = Bundle By Name(cluster=w358, "Synchronize.Echo.Status"="Query Success") -> (w357:T5)
              }
              frame "Revert" {
                n134 = Bundle By Name(cluster=w363, "Synchronize.Echo.Status"="Revert Success") -> (w362:T5)
              }
            }
          }
          frame True {
          }
        }
        n135 = call <vilib>:"Add State(s) to Queue__JKI_lib_State_Machine.vi"("State(s) in Front (\"\")"=w320, "State(s) in (\"\")"=w329) -> ("States Out"=w328:string)  [unwired: 13 in]
      }
      frame "Sync: Release CMD Queue" {
        n136 = Unbundle By Name(w370) -> ("Synchronize.Queue"=w371:refnum<queue>)
        n137 = Release Queue(queue=w371, error in (no error)=w369) -> (error out=w368:errorcluster)  [unwired: 1 in, 2 out]
        n138 = call <vilib>:"Add State(s) to Queue__JKI_lib_State_Machine.vi"("State(s) in (\"\")"=w373) -> ("States Out"=w372:string)  [unwired: 14 in]
      }
      frame "Sync: Send ECHO" {
        n139 = Unbundle By Name(w377) -> ("Synchronize.Communicate"=w374:T10, "Synchronize.EnqueueData.Data"=w386:variant, "Synchronize.Echo"=w378:T12)
        n140 = Variant To Data(error in=w376, type=w374, Variant=w386) -> (data=w379:T10, error out=w380:errorcluster)
        n141 = Unbundle By Name(w379) -> ("ID"=w383:string)
        n142 = Obtain Queue(name (unnamed)=w383, element data type=w378, error in (no error)=w380) -> (queue out=w382:refnum<queue>, error out=w384:errorcluster)  [unwired: 2 in, 1 out]
        n143 = Enqueue Element(queue=w382, element=w378, error in (no error)=w384) -> (queue out=w381:refnum<queue>, error out=w385:errorcluster)  [unwired: 1 in, 1 out]
        n144 = Release Queue(queue=w381, error in (no error)=w385) -> (error out=w375:errorcluster)  [unwired: 1 in, 2 out]
        n145 = call <vilib>:"Add State(s) to Queue__JKI_lib_State_Machine.vi"("State(s) in (\"\")"=w388) -> ("States Out"=w387:string)  [unwired: 14 in]
      }
    }
  }
  n146 = flat-sequence {
    frame #0 {
    }
  }
